vi "Set Input.vi"(10 "Input":variant, 11 "Do Msg in":refnum<class "Do Msg.lvclass">) -> (3 "Do Msg out":refnum<class "Do Msg.lvclass">)   [LabVIEW 2023, in "ITask Actor.lvlib" / "Do Msg.lvclass"]
uses:
  Do Msg.lvclass
  Do Msg.lvclass/Do Msg.ctl
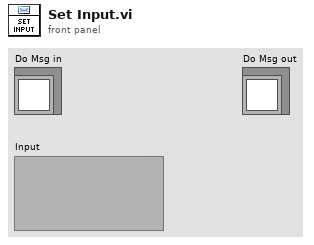
[diagram p1: front panel]
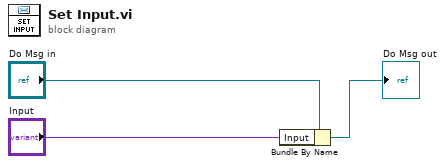
[diagram p0: block diagram]
diagram:
  n1 = Bundle By Name(cluster="Do Msg in", "Input"="Input") -> (→"Do Msg out":refnum<class "Do Msg.lvclass">)
